vi "Login RW.vi"(8 "error in":errorcluster, 9 "Table in":string[][](table)=[["Administrator", "Administrator", "ATS"], ["", "", ""], ["", "", ""]], 10 "Enum":enum16{"write", "read"}(ring)=enum."read", 11 "Path in":path) -> (0 "error out":errorcluster, 2 "Table out":string[][](array[string])=[["Administrator", "Administrator", "ATS"], ["User1", "", ""], ["User2", "", ""]], 3 "Path out":path)   [LabVIEW 2012]
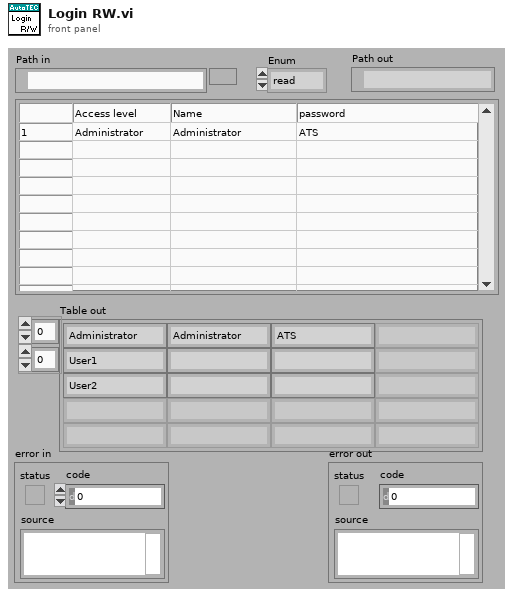
[diagram p1: front panel]
types:
  T1 = enum16{"open", "replace", "create", "open or create", "replace or create", "replace or create with confirmation"}
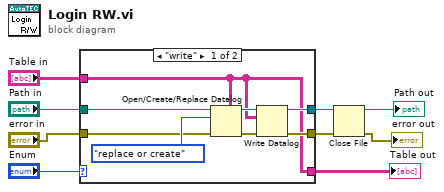
[diagram p0: block diagram]
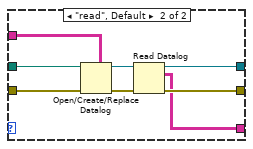
[diagram p2: hidden frame]
diagram:
  n1 = case shown="\"write\"" "Enum" {
    tunnel: [w13 w20] -> w9
    tunnel: [w17 w25] -> w8
    tunnel: [w16 w24] -> w7
    tunnel: "Table in" -> [w13 w22]
    tunnel: "Path in" -> [w15 w23]
    tunnel: "error in" -> [w10 w18]
    frame "write" {
      n2 = Open/Create/Replace Datalog(5:w13, 8:w10, 10:T1."replace or create" ("operation (0:open)"), 11:w15) -> (0:w12:errorcluster, 3:w14:refnum<k1>)  [unwired: 2 in, 1 out]
      n3 = Write Datalog(4:w12, 6:w13, 7:w14) -> (0:w16:errorcluster, 3:w17:refnum<k1>)
    }
    frame "read", Default {
      n4 = Open/Create/Replace Datalog(5:w22, 8:w18, 11:w23) -> (0:w19:errorcluster, 3:w21:refnum<k1>)  [unwired: 3 in, 1 out]
      n5 = Read Datalog(4:w19, 7:w21) -> (0:w24:errorcluster, 2:w20:string[][], 3:w25:refnum<k1>)  [unwired: 1 in]
    }
  }
  "Table out" <- w9
  n6 = Close File(refnum=w8, error in=w7) -> (path=→"Path out":path, error out=→"error out":errorcluster)
